vi "Auto-Refresh Tester.vi"() -> ()   [LabVIEW 2014]
uses:
  DriverMasterSync/build/DriverMasterSync.lvlibp/Modules/HAL/DriverMasterSync/DriverMasterSyncClass/DriverMasterSync.lvclass
  <vilib>/Utility/LVLibp/NI_PackedLibraryUtility.lvlib
panel:
  out "Control Data":T1
  out "1 Sample":cluster{"TDX":sgl[], "TDX Index":u32[]}
  in  "stop":bool
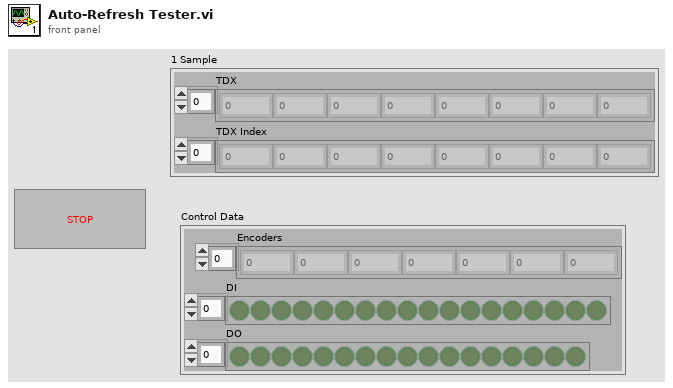
[diagram p1: front panel]
types:
  T1 = cluster{"Encoders":i32[], "DI":bool[], "DO":bool[]}
  T2 = typedef "DriverMasterSync.lvlibp/WINFAS 2 Data Queue.lvlib/Control Data Cluster.ctl" = cluster{"Encoder":sgl, "DI":bool[], "DO":bool[]}
  T3 = typedef "DriverMasterSync.lvlibp/WINFAS 2 Data Queue.lvlib/Acquisition Data 1 Sample Cluster.ctl" = cluster{"TDX":sgl[], "Encoder":sgl}
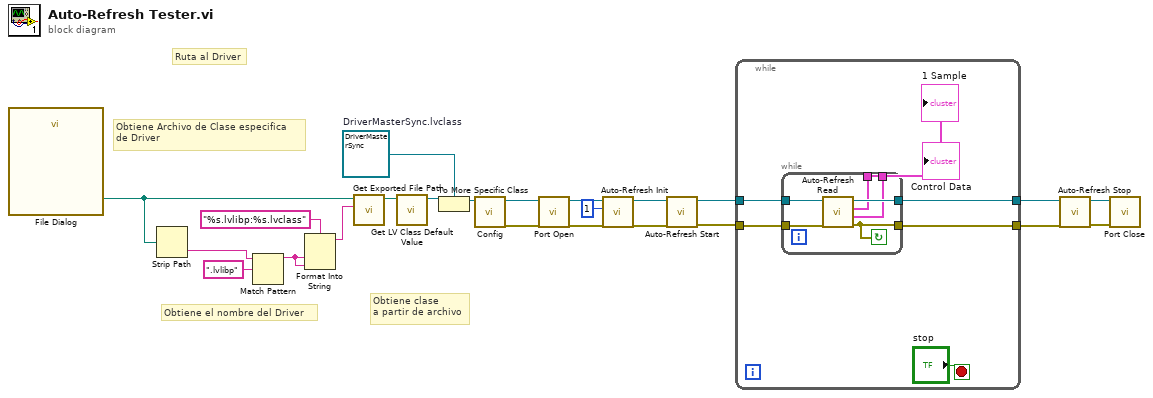
[diagram p0: block diagram]
diagram:
  w6 = refnum<class "DriverMasterSync.lvclass"> refnum  # DriverMasterSync.lvclass
  # "Ruta al Driver"
  # "Obtiene el nombre del Driver"
  # "Obtiene clase\na partir de archivo"
  # "Obtiene Archivo de Clase especifica\nde Driver"
  n1 = call "File Dialog"() -> ("selected path"=w2:path)  [unwired: 12 in, 3 out]
  n2 = Strip Path(path=w2) -> (name=w4:string)  [unwired: 1 out]
  n3 = Match Pattern(string=w4, regular expression=".lvlibp") -> (before substring=w3:string)  [unwired: 1 in, 3 out]
  n4 = Format Into String(format string="%s.lvlibp:%s.lvclass", w3, w3) -> (resulting string=w9:string)  [unwired: 2 in, 1 out]
  n5 = call <vilib>:"Get Exported File Path.vi"("qualified name"=w9, "packed library path"=w2) -> ("path"=w10:path)  [unwired: 8 in, 1 out]
  n6 = call <vilib>:"Get LV Class Default Value.vi"("class path"=w10) -> ("object"=w8:refnum<class>)  [unwired: 9 in, 1 out]
  n7 = To More Specific Class(target class=w6, reference=w8) -> (specific class reference=w1:refnum<class "DriverMasterSync.lvclass">)  [unwired: 1 in, 1 out]
  n8 = call-dynamic "Config.vi"("DriverMasterSync in"=w1) -> ("error out"=w17:errorcluster, "DriverMasterSync out"=w23:refnum<class "DriverMasterSync.lvclass">)  [unwired: 8 in, 1 out]
  n9 = call-dynamic "Port Open.vi"("error in (no error)"=w17, "DriverMasterSync in"=w23) -> ("error out"=w16:errorcluster, "DriverMasterSync out"=w22:refnum<class "DriverMasterSync.lvclass">)  [unwired: 8 in]
  n10 = call-dynamic "Auto-Refresh Init.vi"("error in (no error)"=w16, 10:u64 1 ("Channel Mask"), "DriverMasterSync in"=w22) -> ("error out"=w15:errorcluster, "DriverMasterSync out"=w21:refnum<class "DriverMasterSync.lvclass">)  [unwired: 7 in]
  n11 = call-dynamic "Auto-Refresh Start.vi"("error in (no error)"=w15, "DriverMasterSync in"=w21) -> ("error out"=w14:errorcluster, "DriverMasterSync out"=w20:refnum<class "DriverMasterSync.lvclass">)  [unwired: 8 in]
  n12 = while {
    tunnel: w14 -> [w28]
    tunnel: [w27] -> w13
    tunnel: w20 -> [w30]
    tunnel: [w29] -> w19
    stop <- "stop" stop-if-true
    n13 = while {
      tunnel: [w32] -> w25
      tunnel: [w31] -> w24
      tunnel: w28 -> [w34]
      tunnel: [w33] -> w27
      tunnel: w30 -> [w36]
      tunnel: [w35] -> w29
      stop <- w33 continue-if-true
      n14 = call-dynamic "Auto-Refresh Read.vi"("error in (no error)"=w34, "DriverMasterSync in"=w36) -> ("error out"=w33:errorcluster, "Control Data"=w31:T2, "1 Sample"=w32:T3, "DriverMasterSync out"=w35:refnum<class "DriverMasterSync.lvclass">)  [unwired: 6 in]
    }
    "1 Sample" <- w25
    "Control Data" <- w24
  }
  n15 = call-dynamic "Auto-Refresh Stop.vi"("error in (no error)"=w13, "DriverMasterSync in"=w19) -> ("error out"=w12:errorcluster, "DriverMasterSync out"=w18:refnum<class "DriverMasterSync.lvclass">)  [unwired: 8 in]
  n16 = call-dynamic "Port Close.vi"("error in (no error)"=w12, "DriverMasterSync in"=w18) -> ()  [unwired: 8 in, 2 out]
